vi "Get Error.vi"(11 "Ex Event Actor in":refnum<class "Ex Event Actor.lvclass">) -> (2 "Error":errorcluster)   [LabVIEW 2021, in "Ex Event Actor.lvlib" / "Ex Event Actor.lvclass"]
uses:
  Ex Event Actor.lvclass
  Ex Event Actor.lvclass/Ex Event Actor.ctl
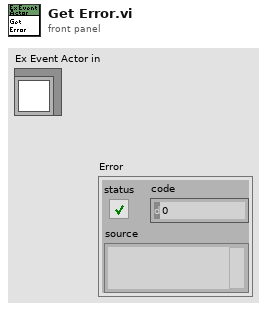
[diagram p1: front panel]
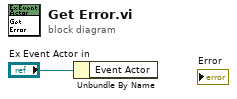
[diagram p0: block diagram]
diagram:
  n1 = Unbundle By Name("Ex Event Actor in") -> ()  [unwired: 1 out]
